vi "TestLtaGet.vi"() -> ()   [LabVIEW 2018, in "Test.lvclass"]
doc: "Tests the retrieval of properties from specific modules (Sensor, AcPwr, Scope, etc)."
uses:
  Test.lvclass
  Test.lvclass/Test.ctl
  Accessors/Write ModuleIDs.vi
panel:
  out "Error Out":errorcluster[](array[cluster])
  in  "ModuleList":string[](array[string])
  in  "ModuleIDs":i32[](array[numeric])
  out "XmlData":string
  in  "Arg":string
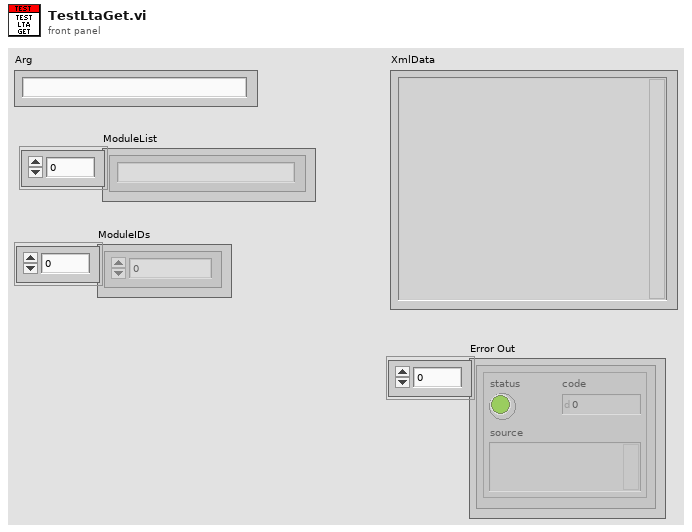
[diagram p1: front panel]
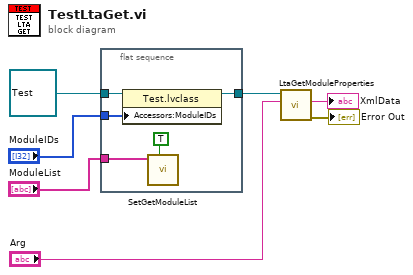
[diagram p0: block diagram]
diagram:
  n1 = flat-sequence {
    tunnel: refnum<class "Test.lvclass"> refnum ("Test.lvclass") -> [w12]
    tunnel: "ModuleIDs" -> [w11]
    tunnel: [w8] -> _
    tunnel: "ModuleList" -> [w10]
    tunnel: [w8] -> w6
    frame #0 {
      n2 = property class="Test.lvclass"(reference=w12, "Accessors:ModuleIDs"=w11) -> (reference out=w8:refnum<class "Test.lvclass">)  [unwired: 1 in, 1 out]
      n3 = call "SetGetModuleList.vi"("Set? (F)"=TRUE ("Set? (f)"), "ModuleList"=w10) -> ()  [unwired: 9 in, 1 out]
    }
  }
  n4 = call "LtaGetModuleProperties.vi"("arg"="Arg", "Test.lvclass"=w6) -> ("Error Out"=→"Error Out":errorcluster[], "XmlData"=→"XmlData":string)  [unwired: 7 in, 1 out]
